vi "Quad_OPC.vi"() -> ()   [LabVIEW 2013]
panel:
  out "URL":string
  out "error out":errorcluster
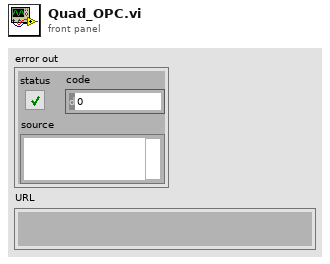
[diagram p1: front panel]
types:
  T1 = enum16{"Read", "Write", "ReadWrite", "BufferedRead", "BufferedReadWrite"}
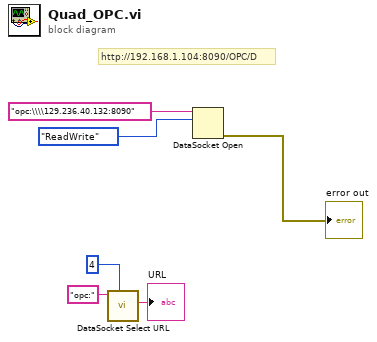
[diagram p0: block diagram]
diagram:
  # "http://192.168.1.104:8090/OPC/D"
  n1 = call <vilib>:"DataSocket Select URL.vi"("Options (0)"=4, "StartURL (empty)"="opc:") -> ("URL"=→"URL":string)  [unwired: 7 in, 2 out]
  n2 = DataSocket Open(10:T1."ReadWrite" ("mode"), 11:"opc:\\\\129.236.40.132:8090" ("URL")) -> (0:→"error out":errorcluster)  [unwired: 2 in, 1 out]
